vi "LOGIC_ChkFrameErr.vi"(8 "error in":errorcluster, 10 "frame status":string) -> (0 "error out":errorcluster)   [LabVIEW 2016]
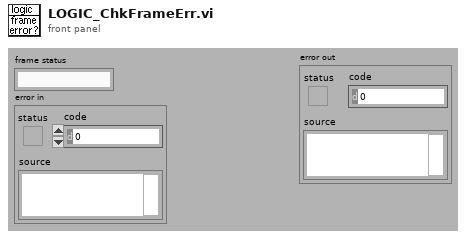
[diagram p1: front panel]
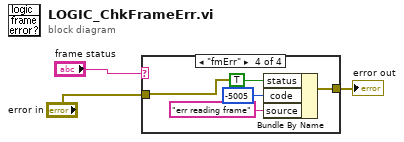
[diagram p0: block diagram]
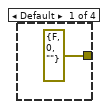
[diagram p2: hidden frame]
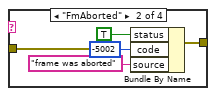
[diagram p3: hidden frame]
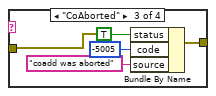
[diagram p4: hidden frame]
diagram:
  n1 = case shown="\"fmErr\"" "frame status" {
    tunnel: "error in" -> [_ w6 w10 w15]
    tunnel: [errorcluster {"status"=FALSE, "code"=0, "source"=""} ("error out") w7 w11 w16] -> w1
    frame Default {
    }
    frame "FmAborted" {
      n2 = Bundle By Name(cluster=w6, "status"=TRUE, "code"=-5002, "source"="frame was aborted") -> (w7:errorcluster)
    }
    frame "CoAborted" {
      n3 = Bundle By Name(cluster=w10, "status"=TRUE, "code"=-5005, "source"="coadd was aborted") -> (w11:errorcluster)
    }
    frame "fmErr" {
      n4 = Bundle By Name(cluster=w15, "status"=TRUE, "code"=-5005, "source"="err reading frame") -> (w16:errorcluster)
    }
  }
  "error out" <- w1
